vi "Actor Core.vi"(8 "error in":errorcluster, 11 "Elevator Controller in":refnum<class "Elevator Controller.lvclass">) -> (0 "error out":errorcluster, 3 "Actor out":refnum<class "Actor.lvclass">)   [LabVIEW 2019, in "Elevator Controller.lvlib" / "Elevator Controller.lvclass"]
doc: "(<B>Filename</B>: Actor Framework.lvlib:Actor.lvclass:Actor Core.vi)\n\nReceives messages to the actor, reacts to them, and initiates any error handling that may shut the actor down.\n\nDescendant classes may override this VI to append parallel tasks for the actor to complete while it handles messages. Overrides use the Call Parent Method node."
uses:
  Elevator Controller.lvclass
  <vilib>/ActorFramework/Actor/Actor.lvclass
  <vilib>/ActorFramework/Stop Msg/Stop Msg.lvclass
  C:/Program Files (x86)/National Instruments/LabVIEW 2019/vi.lib/ActorFramework/Actor/Actor.lvclass
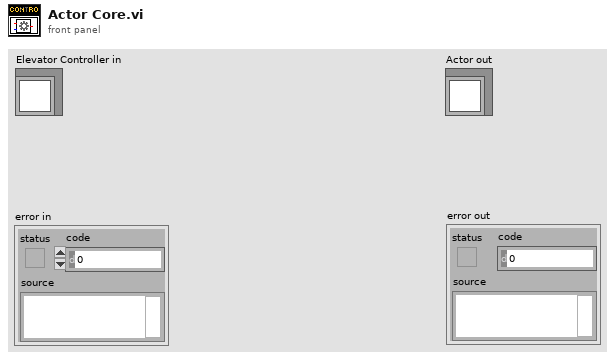
[diagram p1: front panel]
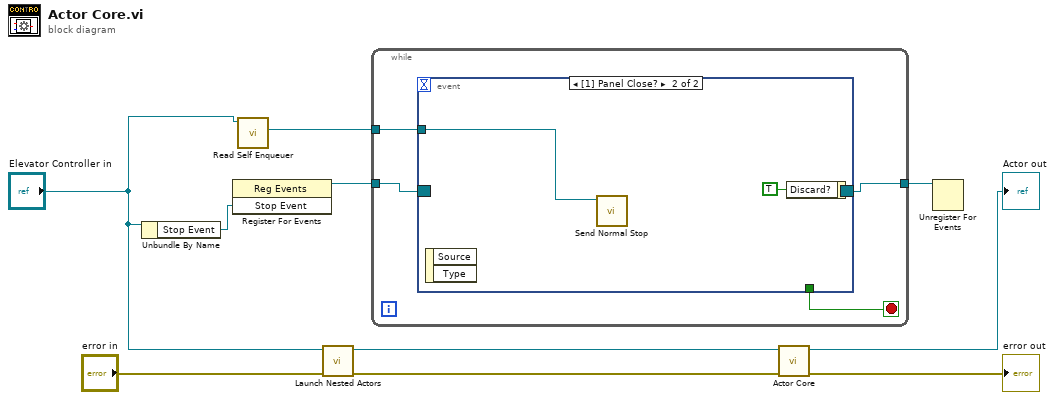
[diagram p0: block diagram]
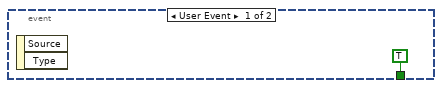
[diagram p2: hidden frame]
diagram:
  n1 = Unbundle By Name("Elevator Controller in") -> ("Stop Event"=w6:refnum<user-event>)
  n2 = register-events(w6) -> (reference out=w8:refnum<event-registration>)  [unwired: 2 in, 1 out]
  n3 = call <vilib>:"Read Self Enqueuer.vi"("Actor"="Elevator Controller in") -> ("Self Enqueuer"=w5:refnum<class "Message Enqueuer.lvclass">)  [unwired: 10 in]
  n4 = call "Launch Nested Actors.vi"("error in (no error)"="error in", "Elevator Controller in"="Elevator Controller in") -> ("error out"=w1:errorcluster, "Elevator Controller out"=w3:refnum<class "Elevator Controller.lvclass">)  [unwired: 8 in]
  n5 = while {
    tunnel: w8 -> [w14]
    tunnel: [w13] -> w7
    tunnel: w5 -> [w12]
    stop <- w11 stop-if-true
    n6 = event shown="[1] Panel Close?" {
      selector: w14 -> [_ _]
      dyn-events: [_ _] -> w13
      timeout: _ -> [_ _]
      tunnel: w12 -> [_ w16]
      tunnel: [TRUE _] -> w11
      event User Event {
        n7 = event-data() -> ()  [unwired: 1 in, 2 out]
      }
      event Panel Close? {
        n8 = event-data() -> ()  [unwired: 1 in, 2 out]
        n9 = call <vilib>:"Send Normal Stop.vi"("Message Enqueuer"=w16) -> ()  [unwired: 10 in, 1 out]
        n10 = event-data("Discard?"=TRUE) -> ()  [unwired: 1 in, 1 out]
      }
    }
  }
  n11 = call-parent "Actor Core.vi"("error in"=w1, "Actor in"=w3) -> ("error out"=→"error out":errorcluster, "Actor out"=→"Actor out":refnum<class "Actor.lvclass">)  [unwired: 8 in]
  n12 = Unregister For Events(event registration refnum=w7) -> ()  [unwired: 1 in, 1 out]
